vi "Create_Request.vi"(6 "Headers":cluster{"Name":string, "Value":string}[](array[cluster]), 8 "error in (no error)":errorcluster, 11 "Base URL":string) -> (0 "error out":errorcluster, 3 "Request out":refnum<class "Request.lvclass">)   [LabVIEW 2016]
uses:
  Request.lvclass
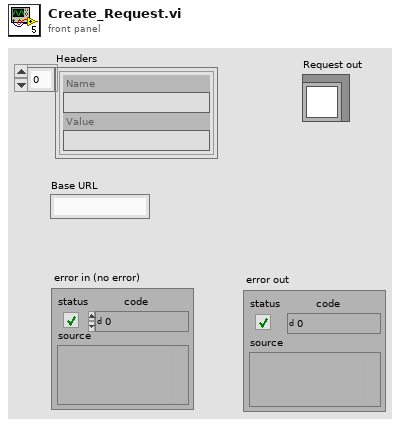
[diagram p1: front panel]
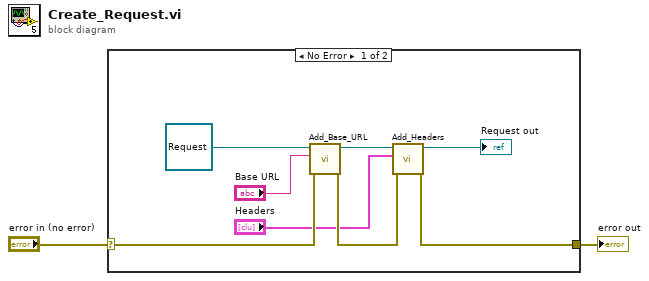
[diagram p0: block diagram]
diagram:
  n1 = case shown="No Error" "error in (no error)" {
    selector: "error in (no error)" -> [w4 w11]
    tunnel: [w5 w11] -> w1
    frame No Error {
      n2 = call "Add_Base_URL.vi"("error in (no error)"=w4, "Base URL"="Base URL", "Request in"=refnum<class "Request.lvclass"> refnum) -> ("error out"=w6:errorcluster, "Request out"=w9:refnum<class "Request.lvclass">)  [unwired: 7 in]
      n3 = call "Add_Headers.vi"("error in (no error)"=w6, "Headers"="Headers", "Request in"=w9) -> ("error out"=w5:errorcluster, "Request out"=→"Request out":refnum<class "Request.lvclass">)  [unwired: 7 in]
    }
    frame Error {
    }
  }
  "error out" <- w1
